vi "Cargo Shoot Control (SubVI).vi"(2 "cargoSensors":T1, 11 "millisecond timer value":u32) -> (3 "shooterInRange":bool, 6 "desiredIntakeOutput":dbl, 8 "desiredIndexerOutput":dbl, 10 "desiredIntakePosition":dbl, 14 "readyToShoot":bool)   [LabVIEW 2020]
uses:
  Cargo Sensors.ctl
  Team Code/Robot Global Data.vi
panel:
  out "hoodInRange":bool
  out "kickupInRange":bool
  out "turretInRange":bool
  out "targetObtained":bool
  in  "hoodTolerance":dbl=20.0
  in  "shooterTolerance":dbl=300.0
  in  "kickupTolerance":dbl=200.0
  in  "turretTolerance":dbl=30.0
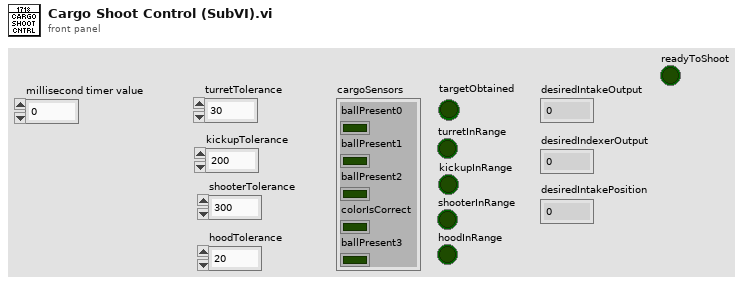
[diagram p1: front panel]
types:
  T1 = typedef "Cargo Sensors.ctl" = cluster{"ballPresent0":bool, "ballPresent1":bool, "ballPresent2":bool, "colorIsCorrect":bool, "ballPresent3":bool}
  T2 = typedef "PiConfig.ctl" = cluster{"swerveModules":cluster{"leftFront":T3, "rightFront":T3, "leftRear":T3, "rightRear":T3}, "offsets":cluster{"leftFrontAngleOffset":dbl, "leftRearAngleOffset":dbl, "rightFrontAngleOffset":dbl, "rightRearAngleOffset":dbl}, "limits":cluster{"maxVelocity":dbl, "maxOverdriveVelocity":dbl, "maxAcceleration":dbl, "maxPickupVelocity":dbl, "maxClimbArmVelocity":dbl}, "speeds":cluster{"intakeSuckSpeed":dbl, "intakeSpitSpeed":dbl, "indexerSuckSpeed":dbl, "indexerSpitSpeed":dbl, "indexerShootSpeed":dbl, "indexerBumpBackSpeed":dbl, "shooterSpinupSpeed":dbl, "kickupSpinupSpeed":dbl, "shooterLowShootSpeed":dbl, "shooterHighShootSpeed":dbl, "shooterPadSpeed":dbl, "shooterWallSpeed":dbl}, "positions":cluster{"intakeStarting":dbl, "intakeStow":dbl, "intakeSuck":dbl, "armPounce":dbl, "armStow":dbl, "armUp":dbl, "winchPounce":dbl, "winchOut":dbl, "winchStow":dbl, "intakeSpit":dbl, "winchBarEngage":dbl, "winchBottomClimb":dbl, "hoodHighShoot":dbl, "armClearHooks":dbl, "winchClearHooks":dbl, "armLiftNextBar":dbl, "winchEngageHooksNextBar":dbl, "winchEngagePassive":dbl, "winchTraversalClimb":dbl, "hoodPadShoot":dbl, "turretPadShoot":dbl, "hoodWallShoot":dbl, "turretWallShoot":dbl, "winchRobotOffBar":dbl, "winchSettleClimb":dbl}, "inversions":cluster{"rightShooter":bool, "leftShooter":bool}}
  T3 = typedef "Swerve Module Parameters.ctl" = cluster{"driveCANID":dbl, "angleCANID":i32, "canCoderCANID":dbl, "moduleName":string, "driveMotorNeutralMode":T4, "driveCurrentLimitConfig":T5, "driveFeedbackDevice":T6, "driveInitialSensorPosition":dbl, "driveEnableVoltageComp":bool, "driveVoltageComp":dbl, "driveRampRate":dbl, "angleCurrentLimit":dbl, "angleSensorType":T7, "angleMotorType":T8, "angleConversionFactor":dbl, "anglePIDRamp":dbl, "angleVoltageComp":dbl, "angleIdleMode":T9, "cancoderConfig":T10, "angleInitialSensorPosition":dbl}
  T4 = typedef "CTRE_Phoenix_MotorControl_NeutralMode.ctl" = enum8{"EEPROMSetting", "Override to Coast", "Override to Brake"}
  T5 = typedef "CTRE_Phoenix_MotorControl_SupplyCurrentLimitConfiguration.ctl" = cluster{"Enable?":bool, "Current Limit":dbl, "Threshold Current":dbl, "Threshold Time":dbl}
  T6 = typedef "CTRE_Phoenix_MotorControl_FeedbackDevice_TalonFX.ctl" = i8
  T7 = typedef "Spark MAX Sensor Type.ctl" = enum16{"No Sensor", "Hall Sensor", "Encoder", "-Not Available-", "Analog", "Alternate Encoder"}
  T8 = typedef "Spark MAX Motor Type.ctl" = enum16{"Brushed", "Brushless"}
  T9 = typedef "Spark MAX Idle Mode.ctl" = enum16{"Coast", "Brake"}
  T10 = typedef "CTRE_Phoenix_CANcoder_Configurables.ctl" = cluster{"Sensor Initialization Strategy":T11, "Absolute Sensor Range":T12, "Velocity Measurement Period":T13, "Velocity Measurement Window":i32, "Magnet Offset (Degrees)":dbl, "Sensor Direction":bool, "Sensor Coefficient":dbl, "Unit String":string, "Sensor Time Base":T14}
  T11 = typedef "CTRE_Phoenix_CANcoder_SensorInitializationStrategy.ctl" = enum16{"Boot To Zero", "Boot To Absolute Position"}
  T12 = typedef "CTRE_Phoenix_CANcoder_AbsoluteSensorRange.ctl" = enum16{"Unsigned [0 to 360)", "Signed [-180 to +180)"}
  T13 = typedef "CTRE_Phoenix_MotorControl_VelocityMeasurementPeriod.ctl" = u16
  T14 = typedef "CTRE_Phoenix_CANcoder_SensorTimeBase.ctl" = enum16{"Per100Ms_Legacy", "PerSecond", "PerMinute"}
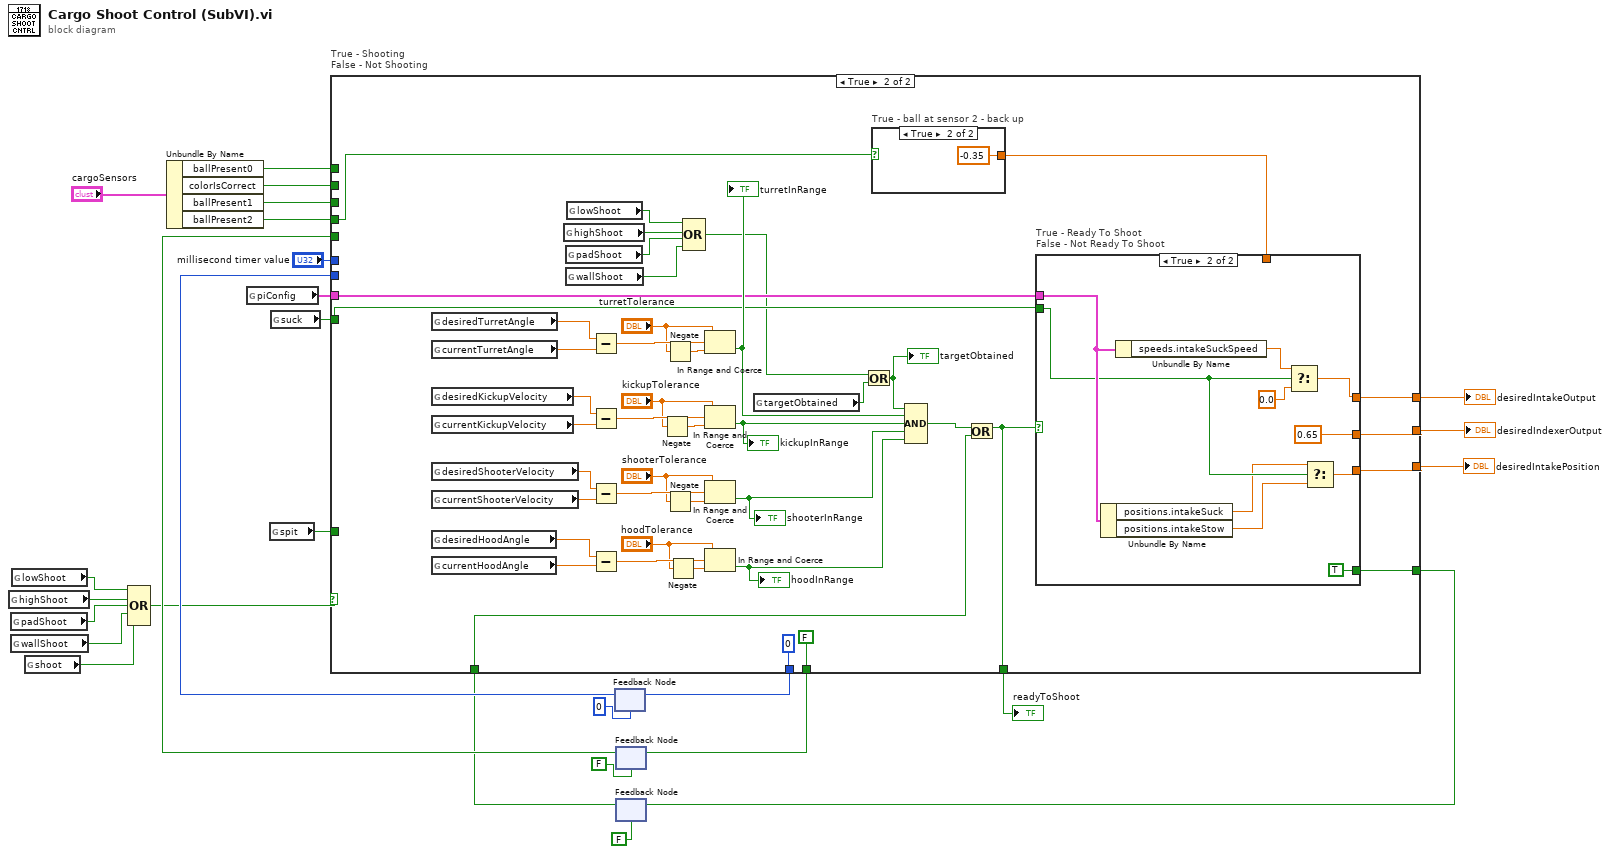
[diagram p0: block diagram]
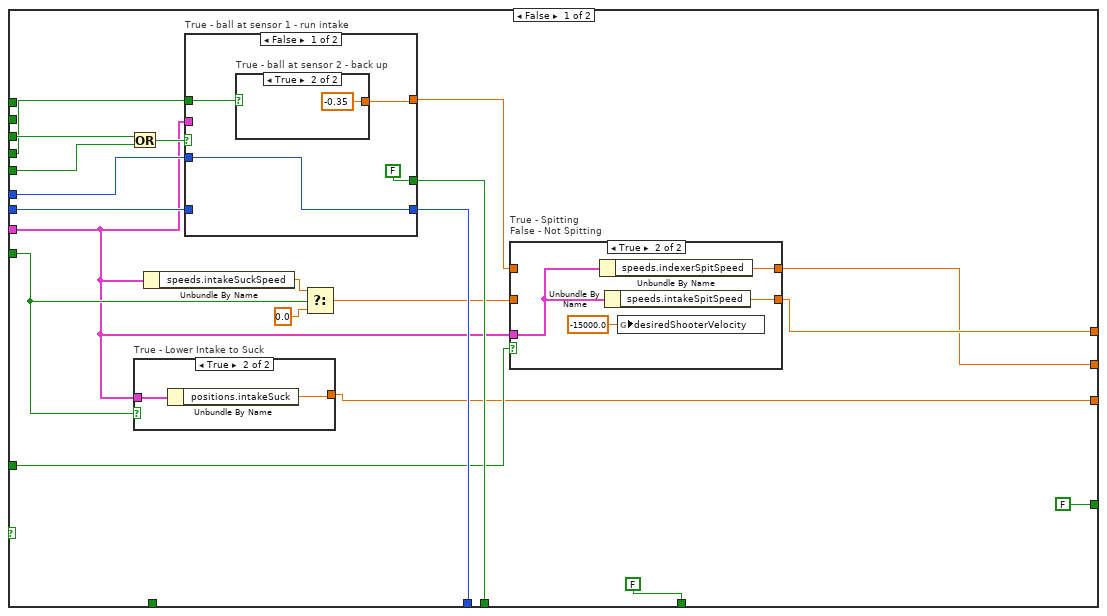
[diagram p2: hidden frame]
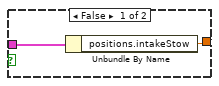
[diagram p3: hidden frame]
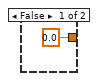
[diagram p5: hidden frame]
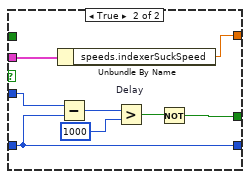
[diagram p6: hidden frame]
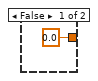
[diagram p7: hidden frame]
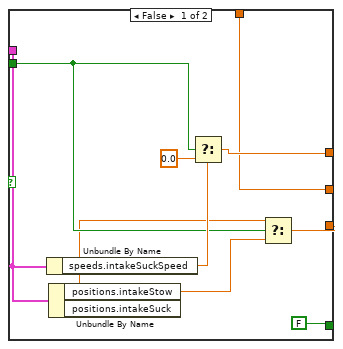
[diagram p8: hidden frame]
diagram:
  n1 = global read "Robot Global Data.vi" "highShoot"() -> (w9:bool)
  n2 = global read "Robot Global Data.vi" "padShoot"() -> (w8:bool)
  n3 = global read "Robot Global Data.vi" "wallShoot"() -> (w7:bool)
  n4 = global read "Robot Global Data.vi" "lowShoot"() -> (w10:bool)
  n5 = global read "Robot Global Data.vi" "shoot"() -> (w4:bool)
  n6 = Compound Arithmetic op=OR(w10, w9, w8, w7, w4) -> (w6:bool)
  n7 = Unbundle By Name("cargoSensors") -> ("ballPresent0"=w11:bool, "colorIsCorrect"=w12:bool, "ballPresent1"=w13:bool, "ballPresent2"=w14:bool)
  n8 = global read "Robot Global Data.vi" "piConfig"() -> (w25:T2)
  n9 = global read "Robot Global Data.vi" "spit"() -> (w24:bool)
  n10 = global read "Robot Global Data.vi" "suck"() -> (w16:bool)
  n11 = feedback #1(u32 0 ("millisecond timer value")) -> (w21:u32)
  n12 = feedback #2(FALSE) -> (w20:bool)
  n13 = feedback #3(FALSE) -> (w1:bool)
  n14 = case "True - Shooting\nFalse - Not Shooting" shown="True" w6 {
    tunnel: w16 -> [w33 w86]
    tunnel: [w39 w115] -> w28
    tunnel: [w37 w116] -> w27
    tunnel: w11 -> [_ _]
    tunnel: w12 -> [_ _]
    tunnel: w13 -> [w46 _]
    tunnel: w14 -> [w34 w78]
    tunnel: "millisecond timer value" -> [w47 _]
    tunnel: w20 -> [w44 _]
    tunnel: w21 -> [w43 _]
    tunnel: [w42 u32 0 ("millisecond timer value")] -> w22
    tunnel: [w41 FALSE] -> w23
    tunnel: w24 -> [w36 _]
    tunnel: w25 -> [w32 w85]
    tunnel: [w31 w84] -> w26
    tunnel: [FALSE w73] -> w5
    tunnel: [FALSE w75] -> w2
    tunnel: w1 -> [_ w74]
    frame False {
      n15 = Or(x=w46, y=w44) -> (x .or. y?=w45:bool)
      n16 = case "True - Lower Intake to Suck" shown="True" w33 {
        tunnel: [w50 w51] -> w31
        tunnel: w32 -> [w49 w52]
        frame False {
          n17 = Unbundle By Name(w49) -> ("positions.intakeStow"=w50:dbl)
        }
        frame True {
          n18 = Unbundle By Name(w52) -> ("positions.intakeSuck"=w51:dbl)
        }
      }
      n19 = Unbundle By Name(w32) -> ("speeds.intakeSuckSpeed"=w35:dbl)
      n20 = case "True - ball at sensor 1 - run intake" shown="False" w45 {
        tunnel: [w59 w66] -> w38
        tunnel: w47 -> [w62 w72]
        tunnel: [w62 w67] -> w42
        tunnel: w43 -> [_ w67]
        tunnel: [FALSE w68] -> w41
        tunnel: w32 -> [_ w65]
        tunnel: w34 -> [w60 _]
        frame False {
          n21 = case "True - ball at sensor 2 - back up" shown="True" w60 {
            tunnel: [0.0 ("s? t:f") -0.35 ("s? t:f")] -> w59
            frame False {
            }
            frame True {
            }
          }
        }
        frame True {
          n22 = Unbundle By Name(w65) -> ("speeds.indexerSuckSpeed"=w66:dbl)
          n23 = Subtract(x=w72, y=w67) -> (x-y=w71:u32)
          n24 = Greater? "Delay"(x=w71, y=u32 1000) -> (0:w69:bool)
          n25 = Not(x=w69) -> (.not. x?=w68:bool)
        }
      }
      n26 = Select(t=w35, s=w33, f=0.0) -> (s? t:f=w40:dbl)
      n27 = case "True - Spitting\nFalse - Not Spitting" shown="True" w36 {
        tunnel: w40 -> [w54 _]
        tunnel: [w54 w58] -> w39
        tunnel: [w53 w57] -> w37
        tunnel: w38 -> [w53 _]
        tunnel: w32 -> [_ w56]
        frame False {
        }
        frame True {
          n28 = Unbundle By Name(w56) -> ("speeds.indexerSpitSpeed"=w57:dbl)
          n29 = Unbundle By Name(w56) -> ("speeds.intakeSpitSpeed"=w58:dbl)
          n30 = global write "Robot Global Data.vi" "desiredShooterVelocity"(-15000.0 ("desiredShooterVelocity")) -> ()
        }
      }
    }
    frame True {
      n31 = global read "Robot Global Data.vi" "desiredTurretAngle"() -> (w91:dbl)
      n32 = global read "Robot Global Data.vi" "currentTurretAngle"() -> (w114:dbl)
      n33 = global read "Robot Global Data.vi" "desiredKickupVelocity"() -> (w110:dbl)
      n34 = global read "Robot Global Data.vi" "currentKickupVelocity"() -> (w109:dbl)
      n35 = global read "Robot Global Data.vi" "desiredShooterVelocity"() -> (w105:dbl)
      n36 = global read "Robot Global Data.vi" "currentShooterVelocity"() -> (w104:dbl)
      n37 = global read "Robot Global Data.vi" "desiredHoodAngle"() -> (w100:dbl)
      n38 = global read "Robot Global Data.vi" "currentHoodAngle"() -> (w99:dbl)
      n39 = global read "Robot Global Data.vi" "highShoot"() -> (w82:bool)
      n40 = global read "Robot Global Data.vi" "padShoot"() -> (w81:bool)
      n41 = global read "Robot Global Data.vi" "wallShoot"() -> (w80:bool)
      n42 = global read "Robot Global Data.vi" "lowShoot"() -> (w83:bool)
      n43 = Subtract(x=w91, y=w114) -> (x-y=w113:dbl)
      n44 = Subtract(x=w110, y=w109) -> (x-y=w108:dbl)
      n45 = Subtract(x=w105, y=w104) -> (x-y=w103:dbl)
      n46 = Subtract(x=w100, y=w99) -> (x-y=w98:dbl)
      n47 = Negate(x="kickupTolerance") -> (-x=w106:dbl)
      n48 = Negate(x="turretTolerance") -> (-x=w111:dbl)
      n49 = Negate(x="shooterTolerance") -> (-x=w101:dbl)
      n50 = Negate(x="hoodTolerance") -> (-x=w96:dbl)
      n51 = Compound Arithmetic op=OR(w83, w82, w81, w80) -> (w79:bool)
      n52 = In Range and Coerce(upper limit="turretTolerance", x=w113, lower limit=w111) -> (In Range?=w95:bool)  [unwired: 1 out]
      "turretInRange" <- w95
      n53 = In Range and Coerce(upper limit="kickupTolerance", x=w108, lower limit=w106) -> (In Range?=w94:bool)  [unwired: 1 out]
      "kickupInRange" <- w94
      n54 = In Range and Coerce(upper limit="shooterTolerance", x=w103, lower limit=w101) -> (In Range?=w93:bool)  [unwired: 1 out]
      "shooterInRange" <- w93
      n55 = In Range and Coerce(upper limit="hoodTolerance", x=w98, lower limit=w96) -> (In Range?=w92:bool)  [unwired: 1 out]
      "hoodInRange" <- w92
      n56 = global read "Robot Global Data.vi" "targetObtained"() -> (w87:bool)
      n57 = Or(x=w79, y=w87) -> (x .or. y?=w88:bool)
      "targetObtained" <- w88
      n58 = case "True - ball at sensor 2 - back up" shown="True" w78 {
        tunnel: [0.0 ("s? t:f") -0.35 ("s? t:f")] -> w77
        frame False {
        }
        frame True {
        }
      }
      n59 = Compound Arithmetic op=AND(w88, w95, w94, w93, w92) -> (w76:bool)
      n60 = Or(x=w76, y=w74) -> (x .or. y?=w73:bool)
      n61 = case "True - Ready To Shoot\nFalse - Not Ready To Shoot" shown="True" w73 {
        tunnel: [w120 0.65 ("Intake")] -> w116
        tunnel: [w127 w134] -> w115
        tunnel: w86 -> [w123 w132]
        tunnel: w85 -> [w128 w137]
        tunnel: [w124 w133] -> w84
        tunnel: w77 -> [w120 _]
        tunnel: [FALSE TRUE] -> w75
        frame False {
          n62 = Unbundle By Name(w128) -> ("speeds.intakeSuckSpeed"=w126:dbl)
          n63 = Unbundle By Name(w128) -> ("positions.intakeStow"=w122:dbl, "positions.intakeSuck"=w121:dbl)
          n64 = Select(t=w126, s=w123, f=0.0) -> (s? t:f=w127:dbl)
          n65 = Select(t=w121, s=w123, f=w122) -> (s? t:f=w124:dbl)
        }
        frame True {
          n66 = Unbundle By Name(w137) -> ("positions.intakeSuck"=w130:dbl, "positions.intakeStow"=w131:dbl)
          n67 = Unbundle By Name(w137) -> ("speeds.intakeSuckSpeed"=w136:dbl)
          n68 = Select(t=w136, s=w132, f=0.0 ("Intake")) -> (s? t:f=w134:dbl)
          n69 = Select(t=w130, s=w132, f=w131) -> (s? t:f=w133:dbl)
        }
      }
    }
  }
  "desiredIntakeOutput" <- w28
  "desiredIndexerOutput" <- w27
  "desiredIntakePosition" <- w26
  "readyToShoot" <- w5
  n70 = feedback-in #1(w22) -> ()
  n71 = feedback-in #2(w23) -> ()
  n72 = feedback-in #3(w2) -> ()
